vi "TWPivotTeleOp.vi"(8 "error in (no error)":errorcluster, 9 "Axes":dbl[](array[numeric]), 10 "Buttons":bool[](array[boolean]), 11 "Robot":T1) -> (0 "error out":errorcluster)   [LabVIEW 2015]
uses:
  Robot Type Def.ctl
  Framework/JoystickMappingNamesTypeDef.ctl
  Lift/TW Global.vi
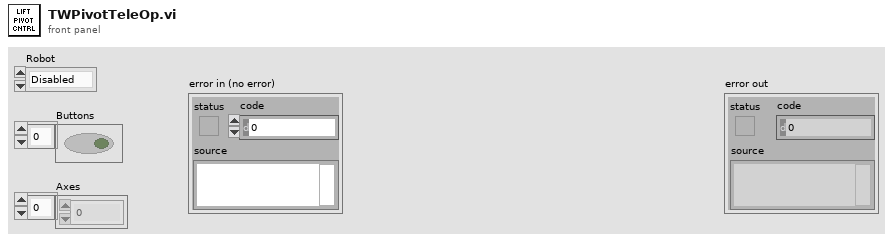
[diagram p1: front panel]
types:
  T1 = typedef "Robot Type Def.ctl" = enum32{"Disabled", "Ghost", "Casper", "Lofty", "Board", "RaceRobot", "Casper 2.0", "Excalibot 2.0"}
  T2 = typedef "JoystickMappingNamesTypeDef.ctl" = enum16{"Shoot Button", "Retrieve Button", "Arm Control", "High Gear", "Low Gear", "Enable PTO", "Disable PTO", "PortC Control", "PortC Up", "PortC Down", "Lift Control", "Drive VBus", "Override Arm Limits", "TWP Control", "TWP Final Pos"}
  T3 = typedef "PortC Settings Type Def.ctl" = cluster{"Down":dbl, "Up":dbl, "Increments":dbl, "Final Pos":dbl}
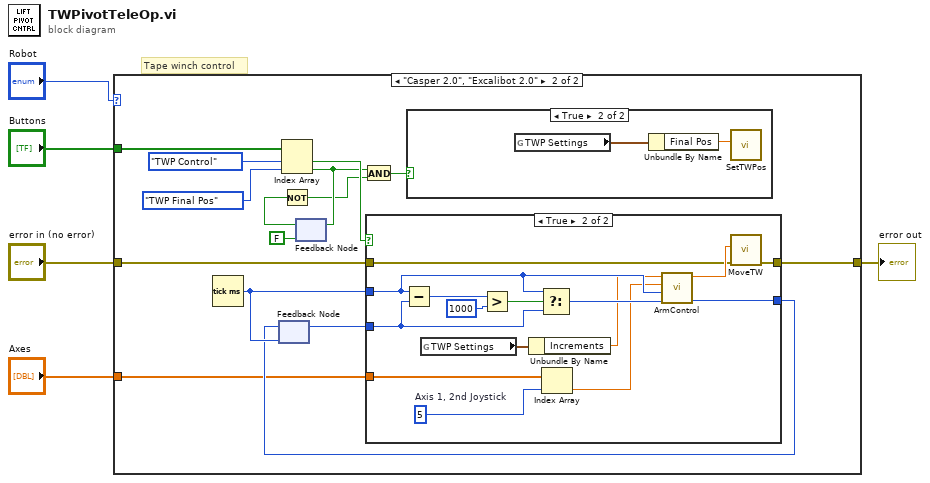
[diagram p0: block diagram]
diagram:
  # "Tape winch control"
  n1 = case shown="\"Casper 2.0\", \"Excalibot 2.0\"" "Robot" {
    tunnel: "Axes" -> [_ w16]
    tunnel: "Buttons" -> [_ w15]
    tunnel: "error in (no error)" -> [w6 w14]
    tunnel: [w6 w13] -> w1
    frame Default {
    }
    frame "Casper 2.0", "Excalibot 2.0" {
      n2 = Tick Count (ms)() -> (millisecond timer value=w21:u32)
      n3 = feedback #1(w21) -> (w20:u32)
      n4 = Index Array(array=w15, index #1=JoystickMappingNamesTypeDef."TWP Control" ("Joystick Button Names"), index #2=JoystickMappingNamesTypeDef."TWP Final Pos" ("Joystick Button Names")) -> (element #1=w18:bool, element #2=w9:bool)
      n5 = feedback #2(FALSE) -> (w11:bool)
      n6 = Not(x=w11) -> (.not. x?=w8:bool)
      n7 = feedback-in #2(w9) -> ()
      n8 = And(x=w9, y=w8) -> (x .and. y?=w10:bool)
      n9 = case shown="True" w18 {
        tunnel: [w25 w35] -> w19
        tunnel: w20 -> [_ w33]
        tunnel: w21 -> [w25 w34]
        tunnel: w16 -> [_ w32]
        tunnel: w14 -> [w24 w28]
        tunnel: [w24 w27] -> w13
        frame False {
        }
        frame True {
          w40 = 5  # Axis 1, 2nd Joystick
          n10 = Subtract(x=w34, y=w33) -> (x-y=w39:u32)
          n11 = global read "TW Global.vi" "TWP Settings"() -> (w31:T3)
          n12 = Greater?(x=w39, y=u32 1000) -> (0:w37:bool)
          n13 = Unbundle By Name(w31) -> ("Increments"=w30:dbl)
          n14 = Select(t=w34, s=w37, f=w33) -> (s? t:f=w36:u32)
          n15 = Index Array(array=w32, index=w40) -> (element=w26:dbl)
          n16 = call "ArmControl.vi"("Last Increment time"=w36, "Current time"=w34, "Joystick"=w26, "Increment"=w30) -> ("Last Time"=w35:u32, "Increment Amount"=w29:dbl)  [unwired: 6 in]
          n17 = call "MoveTW.vi"("error in (no error)"=w28, "Angle"=w29) -> ("error out"=w27:errorcluster)  [unwired: 9 in]
        }
      }
      n18 = feedback-in #1(w19) -> ()
      n19 = case shown="True" w10 {
        frame False {
        }
        frame True {
          n20 = global read "TW Global.vi" "TWP Settings"() -> (w23:T3)
          n21 = Unbundle By Name(w23) -> ("Final Pos"=w22:dbl)
          n22 = call "SetTWPos.vi"("Tick Pos"=w22) -> ()  [unwired: 10 in, 1 out]
        }
      }
    }
  }
  "error out" <- w1
